vi "Add misc test data new.vi"(8 "error in (no error)":errorcluster, 10 "?":T1, 11 "Test in":refnum<k24>) -> (0 "error out":errorcluster, 3 "Test out":refnum<k24>)   [LabVIEW 2018]
uses:
  C:/Program Files (x86)/National Instruments/LabVIEW 2018/user.lib/nEQdb_DLL/NEQdbAPI.dll
  Program Files (x86)/National Instruments/LabVIEW 2018/user.lib/nEQdb_DLL/NEQdbAPI.dll
  State data/Records.ctl
panel:
  in  "Enum":T2(ring)
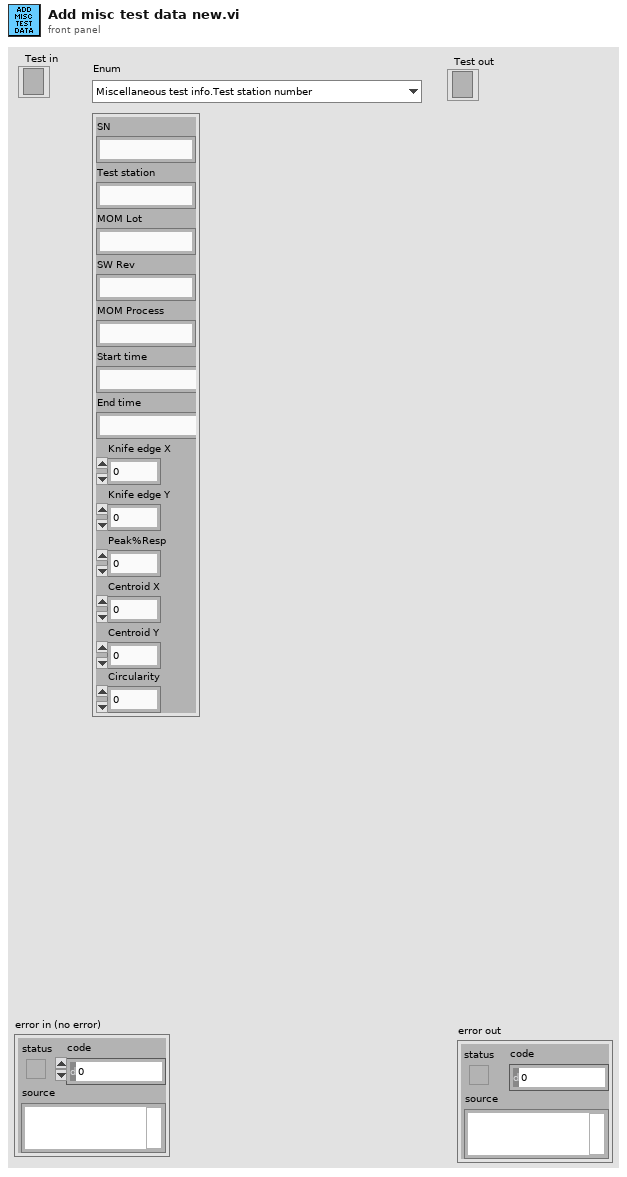
[diagram p1: front panel]
types:
  T1 = typedef "Records.ctl" = cluster{"SN":string, "Test station":string, "MOM Lot":string, "SW Rev":string, "MOM Process":string, "Start time":string, "End time":string, "Knife edge X":dbl, "Peak%Resp":dbl, "Centroid X":dbl, "Knife edge Y":dbl, "Centroid Y":dbl, "Circularity":dbl}
  T2 = enum16{"Miscellaneous test info.Test station number", "Miscellaneous test info.Software version", "MOM info.LotID", "MOM info.Process step name"}
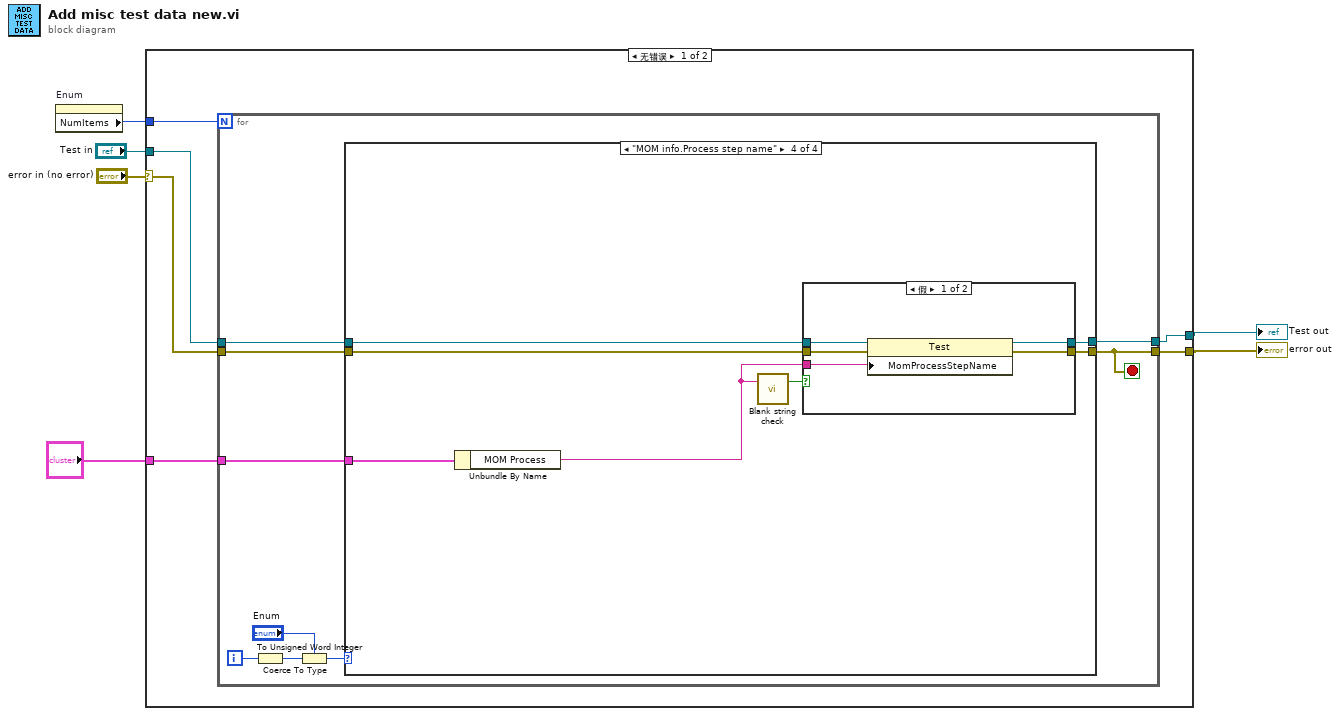
[diagram p0: block diagram]
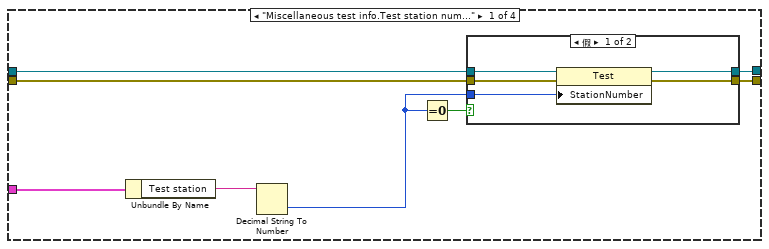
[diagram p2: hidden frame]
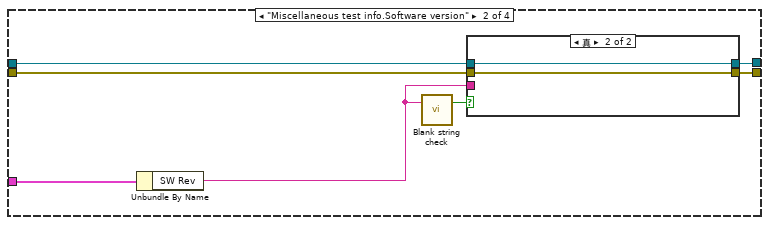
[diagram p4: hidden frame]
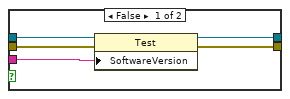
[diagram p5: hidden frame]
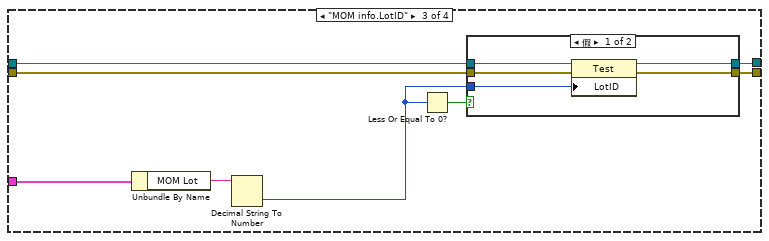
[diagram p6: hidden frame]
diagram:
  n1 = property on="Enum" class="Enum (严格)"() -> ("NumItems"=w4:u32)  [unwired: 2 in, 2 out]
  n2 = case shown="无错误" "error in (no error)" {
    selector: "error in (no error)" -> [w8 w81]
    tunnel: [w12 w81] -> w2
    tunnel: "?" -> [w11 _]
    tunnel: "Test in" -> [w10 w80]
    tunnel: [w9 w80] -> w3
    tunnel: w4 -> [w7 _]
    frame No Error {
      n3 = for {
        N: w7 -> [_]
        tunnel: w11 -> [w17]
        tunnel: w8 -> [w16]
        tunnel: w10 -> [w15]
        tunnel: [w14] -> w9
        tunnel: [w13] -> w12
        i -> [w21]
        stop <- w13 stop-if-true
        n4 = To Unsigned Word Integer(number=w21) -> (unsigned 16bit integer=w20:u16)
        n5 = Coerce To Type(0:w20, 1:"Enum") -> (2:w18:T2)
        n6 = case shown="\"MOM info.Process step name\"" w18 {
          tunnel: w17 -> [w29 w43 w58 w72]
          tunnel: w16 -> [w27 w41 w56 w70]
          tunnel: w15 -> [w28 w42 w57 w71]
          tunnel: [w26 w40 w55 w69] -> w13
          tunnel: [w25 w39 w54 w68] -> w14
          frame "Miscellaneous test info.Test station number" {
            n7 = Unbundle By Name(w29) -> ("Test station"=w23:string)
            n8 = Decimal String To Number(string=w23) -> (number=w22:i32)  [unwired: 2 in, 1 out]
            n9 = Equal To 0?(x=w22) -> (x = 0?=w24:bool)
            n10 = case shown="假" w24 {
              tunnel: w22 -> [w34 _]
              tunnel: w27 -> [w33 w35]
              tunnel: w28 -> [w32 w36]
              tunnel: [w31 w35] -> w26
              tunnel: [w30 w36] -> w25
              frame False {
                n11 = property class="Test"(reference=w32, error in=w33, "StationNumber"=w34) -> (reference out=w30:refnum<k24>, error out=w31:errorcluster)
              }
              frame True {
              }
            }
          }
          frame "Miscellaneous test info.Software version" {
            n12 = Unbundle By Name(w43) -> ("SW Rev"=w37:string)
            n13 = call <userlib>:"Blank string check.vi"("String for nEQdb"=w37) -> ("Blank or NaN?"=w38:bool)  [unwired: 2 in]
            n14 = case shown="真" w38 {
              tunnel: w37 -> [w48 _]
              tunnel: w41 -> [w47 w49]
              tunnel: w42 -> [w46 w50]
              tunnel: [w45 w49] -> w40
              tunnel: [w44 w50] -> w39
              frame False {
                n15 = property class="Test"(reference=w46, error in=w47, "SoftwareVersion"=w48) -> (reference out=w44:refnum<k24>, error out=w45:errorcluster)
              }
              frame True {
              }
            }
          }
          frame "MOM info.LotID" {
            n16 = Unbundle By Name(w58) -> ("MOM Lot"=w52:string)
            n17 = Decimal String To Number(string=w52) -> (number=w51:i32)  [unwired: 2 in, 1 out]
            n18 = Less Or Equal To 0?(x=w51) -> (x <= 0?=w53:bool)
            n19 = case shown="假" w53 {
              tunnel: w51 -> [w63 _]
              tunnel: w56 -> [w62 w64]
              tunnel: w57 -> [w61 w65]
              tunnel: [w60 w64] -> w55
              tunnel: [w59 w65] -> w54
              frame False {
                n20 = property class="Test"(reference=w61, error in=w62, "LotID"=w63) -> (reference out=w59:refnum<k24>, error out=w60:errorcluster)
              }
              frame True {
              }
            }
          }
          frame "MOM info.Process step name" {
            n21 = Unbundle By Name(w72) -> ("MOM Process"=w67:string)
            n22 = call <userlib>:"Blank string check.vi"("String for nEQdb"=w67) -> ("Blank or NaN?"=w66:bool)  [unwired: 2 in]
            n23 = case shown="假" w66 {
              tunnel: w70 -> [w77 w78]
              tunnel: w71 -> [w76 w79]
              tunnel: [w75 w78] -> w69
              tunnel: [w74 w79] -> w68
              tunnel: w67 -> [w73 _]
              frame False {
                n24 = property class="Test"(reference=w76, error in=w77, "MomProcessStepName"=w73) -> (reference out=w74:refnum<k24>, error out=w75:errorcluster)
              }
              frame True {
              }
            }
          }
        }
      }
    }
    frame Error {
    }
  }
  "error out" <- w2
  "Test out" <- w3
